vi "PPMS2_Sort.vi"(8 "pattern":string="ppms2log*dat", 9 "directory path":path=path "\\\\PPMS2\\Data/PPMS Log") -> (2 "Array":string[](array[string]))   [LabVIEW 2016]
panel:
  # "List files in a specified folder in order of time stamp.\n\nDaniel L. Press\nPrimeTest Corp.\ndan.press@primetest.com"
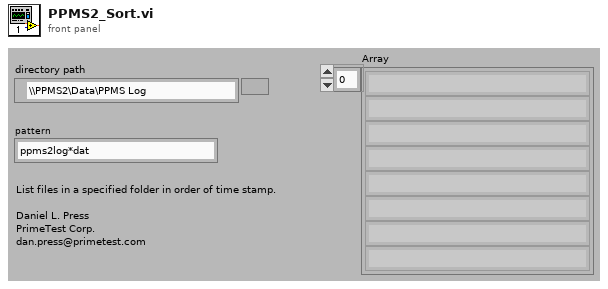
[diagram p1: front panel]
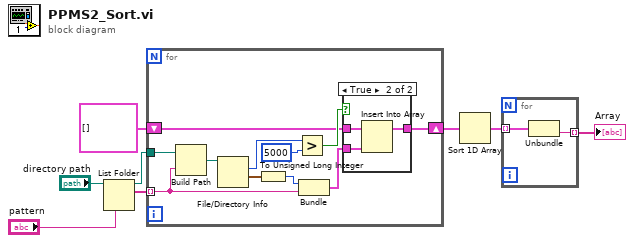
[diagram p0: block diagram]
diagram:
  n1 = List Folder(path="directory path", pattern="pattern") -> (path out=w7:path, filenames=w8:string[])  [unwired: 2 in, 2 out]
  n2 = for {
    tunnel: w8 -> [w16] mode=indexing
    tunnel: w7 -> [w19]
    shift-right: [w10] -> w6
    shift-left: cluster{u32, string}[] [] -> [w9]
    n3 = Build Path(base path=w19, name or relative path=w16) -> (appended path=w17:path)
    n4 = File/Directory Info(path=w17) -> (size=w14:i64, last mod=w15:timestamp)  [unwired: 1 in, 5 out]
    n5 = To Unsigned Long Integer(number=w15) -> (unsigned 32bit integer=w18:u32)
    n6 = Greater?(x=w14, y=i64 5000) -> (0:w12:bool)
    n7 = Bundle(w18, w16) -> (w11:cluster{u32, string})  [unwired: 1 in]
    n8 = case shown="True" w12 {
      tunnel: w11 -> [_ w23]
      tunnel: [w20 w22] -> w10
      tunnel: w9 -> [w20 w21]
      frame False {
      }
      frame True {
        n9 = Insert Into Array(array=w21, new element=w23) -> (w22:cluster{u32, string}[])  [unwired: 1 in]
      }
    }
  }
  n10 = Sort 1D Array(array=w6) -> (sorted array=w3:cluster{u32, string}[])
  n11 = for {
    tunnel: w3 -> [w25] mode=indexing
    tunnel: [w24] -> w2 mode=indexing
    n12 = Unbundle(w25) -> (w24:string)  [unwired: 1 out]
  }
  "Array" <- w2
